vi "Dashboard Main.vi"() -> ()   [LabVIEW 2019]
uses:
  <vilib>/Utility/miscctls.llb/LVRowAndColumnTypeDef.ctl
  <vilib>/event_ctls.llb/eventvkey.ctl
  <vilib>/Rock Robotics/Network Tables/NT Read Numeric Array.vi
  <vilib>/Rock Robotics/WPI/Dashboard/WPI_DashboardLogging Global.vi
  <vilib>/Rock Robotics/Network Tables/NT Read Boolean.vi
panel:
  in  "Camera Settings Right":T1={"Frame Rate"=30, "Compression"=30, "Size"=1, "DB Camera Config"=FALSE} {"Frame Rate" scale=1.0..30.0; "Compression" scale=100.0..-1.0; "Size" items=["640x480", "320x240", "160x120"]}
  in  "Camera Name Right":string(combo)="No Camera Selection"
  out "Camera Perf":string
  in  "Camera Settings":T1={"Frame Rate"=30, "Compression"=30, "Size"=1, "DB Camera Config"=FALSE} {"Frame Rate" scale=1.0..30.0; "Compression" scale=100.0..-1.0; "Size" items=["640x480", "320x240", "160x120"]}
  in  "TCP":refnum<k5>
  in  "Rec Mode":enum32{"Stop", "Record", "Playback"}(radio)
  out "Robot IP":string
  out "Image Message":string="Timeout in Camera Communications"
  in  "Dashboard Tab":T2(tab)
  in  "Select Auto":string(combo)="Select Autonomous ..."
  out "NT Connection":bool
  out "MotorChart R":cluster{"Numeric":dbl, "Numeric":dbl}(graph)
  out "MotorChart L":cluster{"Numeric":dbl, "Numeric":dbl}(graph)
  out "MotorSliders R":cluster{"MotorSlide1":dbl, "MotorSlide2":dbl} {"MotorSlide2" scale=-1.0..1.0 scale format="%#_2e"; "MotorSlide1" scale=-1.0..1.0 scale format="%#_2e"}
  out "MotorSliders L":cluster{"MotorSlide1":dbl, "MotorSlide2":dbl} {"MotorSlide2" scale=-1.0..1.0 scale format="%#_2e"; "MotorSlide1" scale=-1.0..1.0 scale format="%#_2e"}
  out "Gyro":dbl(knob) scale=0.0..360.0
  out "JS1 Z":dbl(slide) scale=-1.0..1.0 scale format="%#_2e"
  out "JS1 Graph":cluster{"X":dbl, "Y":dbl}[](graph)
  out "JS1 Buttons":T3
  out "JS2 Z":dbl(slide) scale=-1.0..1.0 scale format="%#_2e"
  out "JS2 Graph":cluster{"X":dbl, "Y":dbl}[](graph)
  out "JS2 Buttons":T3
  out "Mode":T4(ring)=enum."Auto Disabled"
  out "Right Camera Perf":cluster{"Bandwidth (Mbps)":dbl, "FPS":dbl}
  out "Ball Intake":dbl
  out "Camera Image Right":T5(plugin-control)
  in  "DB/String 9":string
  in  "DB/String 8":string
  in  "DB/String 7":string
  in  "DB/String 6":string
  in  "DB/String 5":string
  in  "DB/String 4":string
  in  "DB/String 3":string
  in  "DB/String 2":string
  in  "DB/String 1":string
  in  "DB/String 0":string
  in  "DB/Slider 0":dbl(slide) scale=0.0..5.0
  in  "DB/Slider 1":dbl(slide) scale=0.0..5.0
  in  "DB/Slider 2":dbl(slide) scale=0.0..5.0
  in  "DB/Slider 3":dbl(slide) scale=0.0..5.0
  out "DB/LED 3":bool
  out "DB/LED 2":bool
  out "DB/LED 1":bool
  out "DB/LED 0":bool
  in  "DB/Button 3":bool
  in  "DB/Button 2":bool
  in  "DB/Button 1":bool
  in  "DB/Button 0":bool caption="New Name"
  out "Touching?":bool
  out "Color":u32(colorbox)
  out "Color Name":string
  out "Proximity":dbl
  out "Confidence":dbl
  in  "Test Slider":dbl(slide) scale=0.0..100.0 scale format="%#_3g"
  in  "On/Off":bool caption="Solenoid"
  in  "Test Name":u16(ring) items=["Select the test to run..."]
  in  "Test Tree":string(tree)
  in  "Motor":cluster{"Value":dbl, "Enable":bool} {"Value" scale=-1.0..1.0 scale format="%#_3g"}
  out "Progress":T6 {"Test Progress" scale=0.0..100.0}
  in  "Rev/Fwd":cluster{"Forward":bool, "Reverse":bool}
  in  "Test Ring":u16(ring) items=["Monochrome", "Color"]
  out "Cmd Status":string
  in  "Execute Command":bool
  in  "Command Params":string[][](table)
  in  "Command Selection":i32(listbox)
  in  "CheckList":i32(listbox)
  out "Tree":string(tree)
  out "Camera Image":T5(plugin-control)
  out "Background":bool
  in  "Camera Name":string(combo)="No Camera Selection"
  # "HW"
  # "HW"
  # "Joysticks"
  # "Drive Motors"
  # "Front"
  # "Right"
  # "Left"
  # "Back"
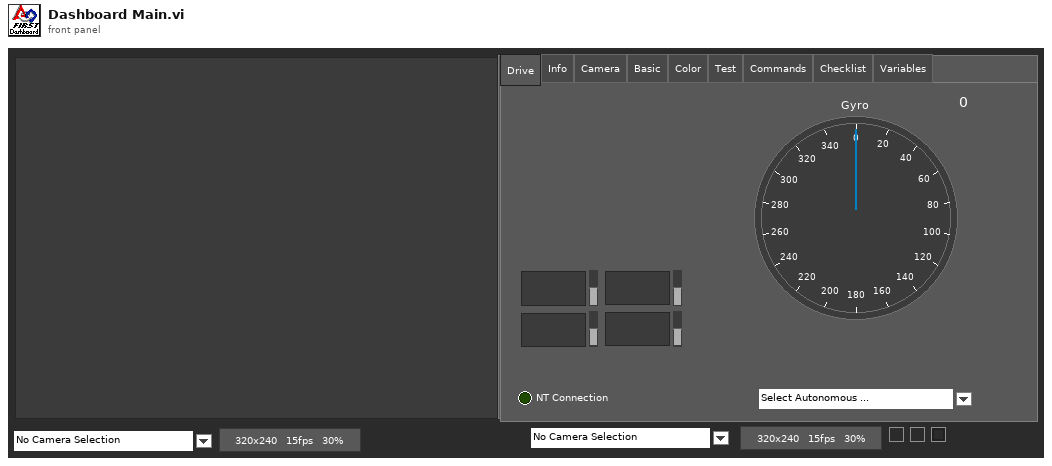
[diagram p1: front panel]
types:
  T1 = cluster{"Frame Rate":i32, "Compression":i32, "Size":u16, "DB Camera Config":bool}
  T2 = enum32{"Drive", "Info", "Camera", "Basic", "Color", "Test", "Commands", "Checklist", "Variables"}
  T3 = cluster{bool, bool, bool, bool, bool, bool, bool, bool, bool, bool, bool, bool}
  T4 = enum8{"Tele-Op Disabled", "Tele-Op Enabled", "Auto Disabled", "Auto Enabled", "Test Disabled", "Test Enabled", "Disconnected", "No Code", "E-Stop"}
  T5 = typedef "IMAQ Image.ctl" = refnum<image>
  T6 = cluster{"Test Progress":u8, "Test Progress Text":string}
  T7 = cluster{"Save Path":path, "Interval (s)":dbl, "Keep":i32}
  T8 = enum32{"Drive", "Camera", "Basic", "Custom", "Test", "Commands", "Checklist", "Variables"}
  T9 = typedef "Image Type" = u32
  T10 = cluster{"IDs":cluster{"RPC field ID":u16, "Unique ID":u16}, "String":string}
  T11 = cluster{"Error Strings":string, "Disable Counts":cluster{u16, u16}, "Rail Faults":cluster{u16, u16, u16}, "Robot IP":string, "DB Mode":u8, "Event Info":cluster{"Name":string, "Type":u8, "Number":u16, "Replay":u8}}
  T12 = cluster{"Storage":cluster{"Disk Free":u64, "RAM Block":u32, "RAM free":u32}, "CPU Utilization":cluster{"CPU % ISR":sgl, "CPU % Time Crit":sgl, "CPU % Timed Str":sgl, "CPU % High":sgl, "CPU % Above":sgl, "CPU % Normal":sgl, "CPU % Low":sgl}, "CAN":cluster{"% Bus Utilization":sgl, "Bus Off Cnt":u32, "TX_FIFO Full Cnt":u32, "Receive Error Cnt":u8, "Transmit Error Cnt":u8}, "HID":cluster{"HID Outputs":u32, "Rumble Low":u16, "Rumble High":u16}[]}
  T13 = cluster{"Status bits":cluster{"Test Mode":bool, "Autonomous":bool, "Enabled":bool, "Code Start":bool, "Brownout":bool, "Reserved 2":bool, "Reserved 3":bool, "E-Stop":bool}, "Code Trace":cluster{"Disabled":bool, "TeleOp":bool, "Auto":bool, "Test":bool}, "Controller Type":enum16{"unknown", "cRIO", "roboRio"}, "Code?":enum16{"unknown", "noCode", "code"}, "Battery V":dbl}
  T14 = cluster{"Control Bits":cluster{"TestMode":bool, "Autonomous":bool, "Enabled":bool, "FMS Present":bool, bool, bool, bool, "E-Stop":bool}, "Team Station ":u8, "Countdown":sgl, "Joystick Values":cluster{"Axes":dbl[], "Buttons":bool[], "POVs":i16[]}[]}
  T15 = cluster{"Axes":dbl[], "Buttons":bool[], "POVs":i16[]}[]
  T16 = cluster{"Axes":dbl[], "Buttons":bool[], "POVs":i16[]}
  T17 = cluster{"Buttons[0]":bool, "Buttons[1]":bool, "Buttons[2]":bool, "Buttons[3]":bool, "Buttons[4]":bool, "Buttons[5]":bool, "Buttons[6]":bool, "Buttons[7]":bool, "Buttons[8]":bool, "Buttons[9]":bool, "Buttons[10]":bool, "Buttons[11]":bool}
  T18 = cluster{"Camera Image":refnum<vi>, "Dashboard Tab":refnum<vi>, "Background":refnum<vi>, "Rec Mode":refnum<vi>, "Test Slider":refnum<vi>, "On/Off ":refnum<vi>, "Test Ring":refnum<vi>, "Rev/Fwd":refnum<vi>, "Test Name":refnum<vi>, "Motor":refnum<vi>, "Progress":refnum<vi>, "CheckList":refnum<vi>, "Tree":refnum<vi>, "Test Tree":refnum<vi>, "Command Params":refnum<vi>, "Command Selection":refnum<vi>, "Execute Command":refnum<vi>, "Cmd Status":refnum<vi>, "Camera Settings":refnum<vi>, "Camera Name":refnum<vi>, "Camera Perf":refnum<vi>, "Camera Settings Right":refnum<vi>, "Camera Name Right":refnum<vi>, "Camera Image Right":refnum<vi>}
  T19 = cluster{"Global Rectangle":i32[], "Contours":cluster{"Contour Type":u32, "ROI Type":u32, "Points":i32[]}[]}
  T20 = cluster{"Camera Name":string, string, "Saved DB Images Info":cluster{"Save Path":path, "Interval (s)":dbl, "Keep":i32}}
  T21 = cluster{"Camera Name Right":string, string, "Saved DB Images Info":cluster{"Save Path":path, "Interval (s)":dbl, "Keep":i32}}
  T22 = cluster{"Operation":enum16{"Update", "Clear"}, "Color Box":u32}[]
  T23 = typedef "eventvkey.ctl" = enum16{"ASCII", "Enter", "Return", "Shift", "Ctrl", "Alt", "Cmd", "Opt", "Caps", "NumLock", "Clear", "Break", "Up", "Down", "Left", "Right", "Insert", "Delete", "Home", "End", "PageUp", "PageDown", "Escape", "Help", "Pause", "ScrollLock", "F1", "F2", "F3", "F4", "F5", "F6", "F7", "F8", "F9", "F10", "F11", "F12", "F13", "F14", "F15", "F16", "F17", "F18", "F19", "F20", "F21", "F22", "F23", "F24", "Play", "VolumeUp", "VolumeDown", "Mute", "Two Byte Char"}
  T24 = cluster{"Image Size":bool, "Image Type":bool, "Pixel Value":bool, "ROI Information":bool, "Zoom Factor":bool}
  T25 = cluster{"Operation":enum16{"Update", "Clear"}, "Color Box":u32}
  T26 = typedef "LVRowAndColumnTypeDef.ctl" = cluster{"Row":i32, "Column":i32}
  T27 = cluster{"Shift":bool, "Ctrl":bool, "Alt":bool, "Cmd":bool, "Opt":bool}
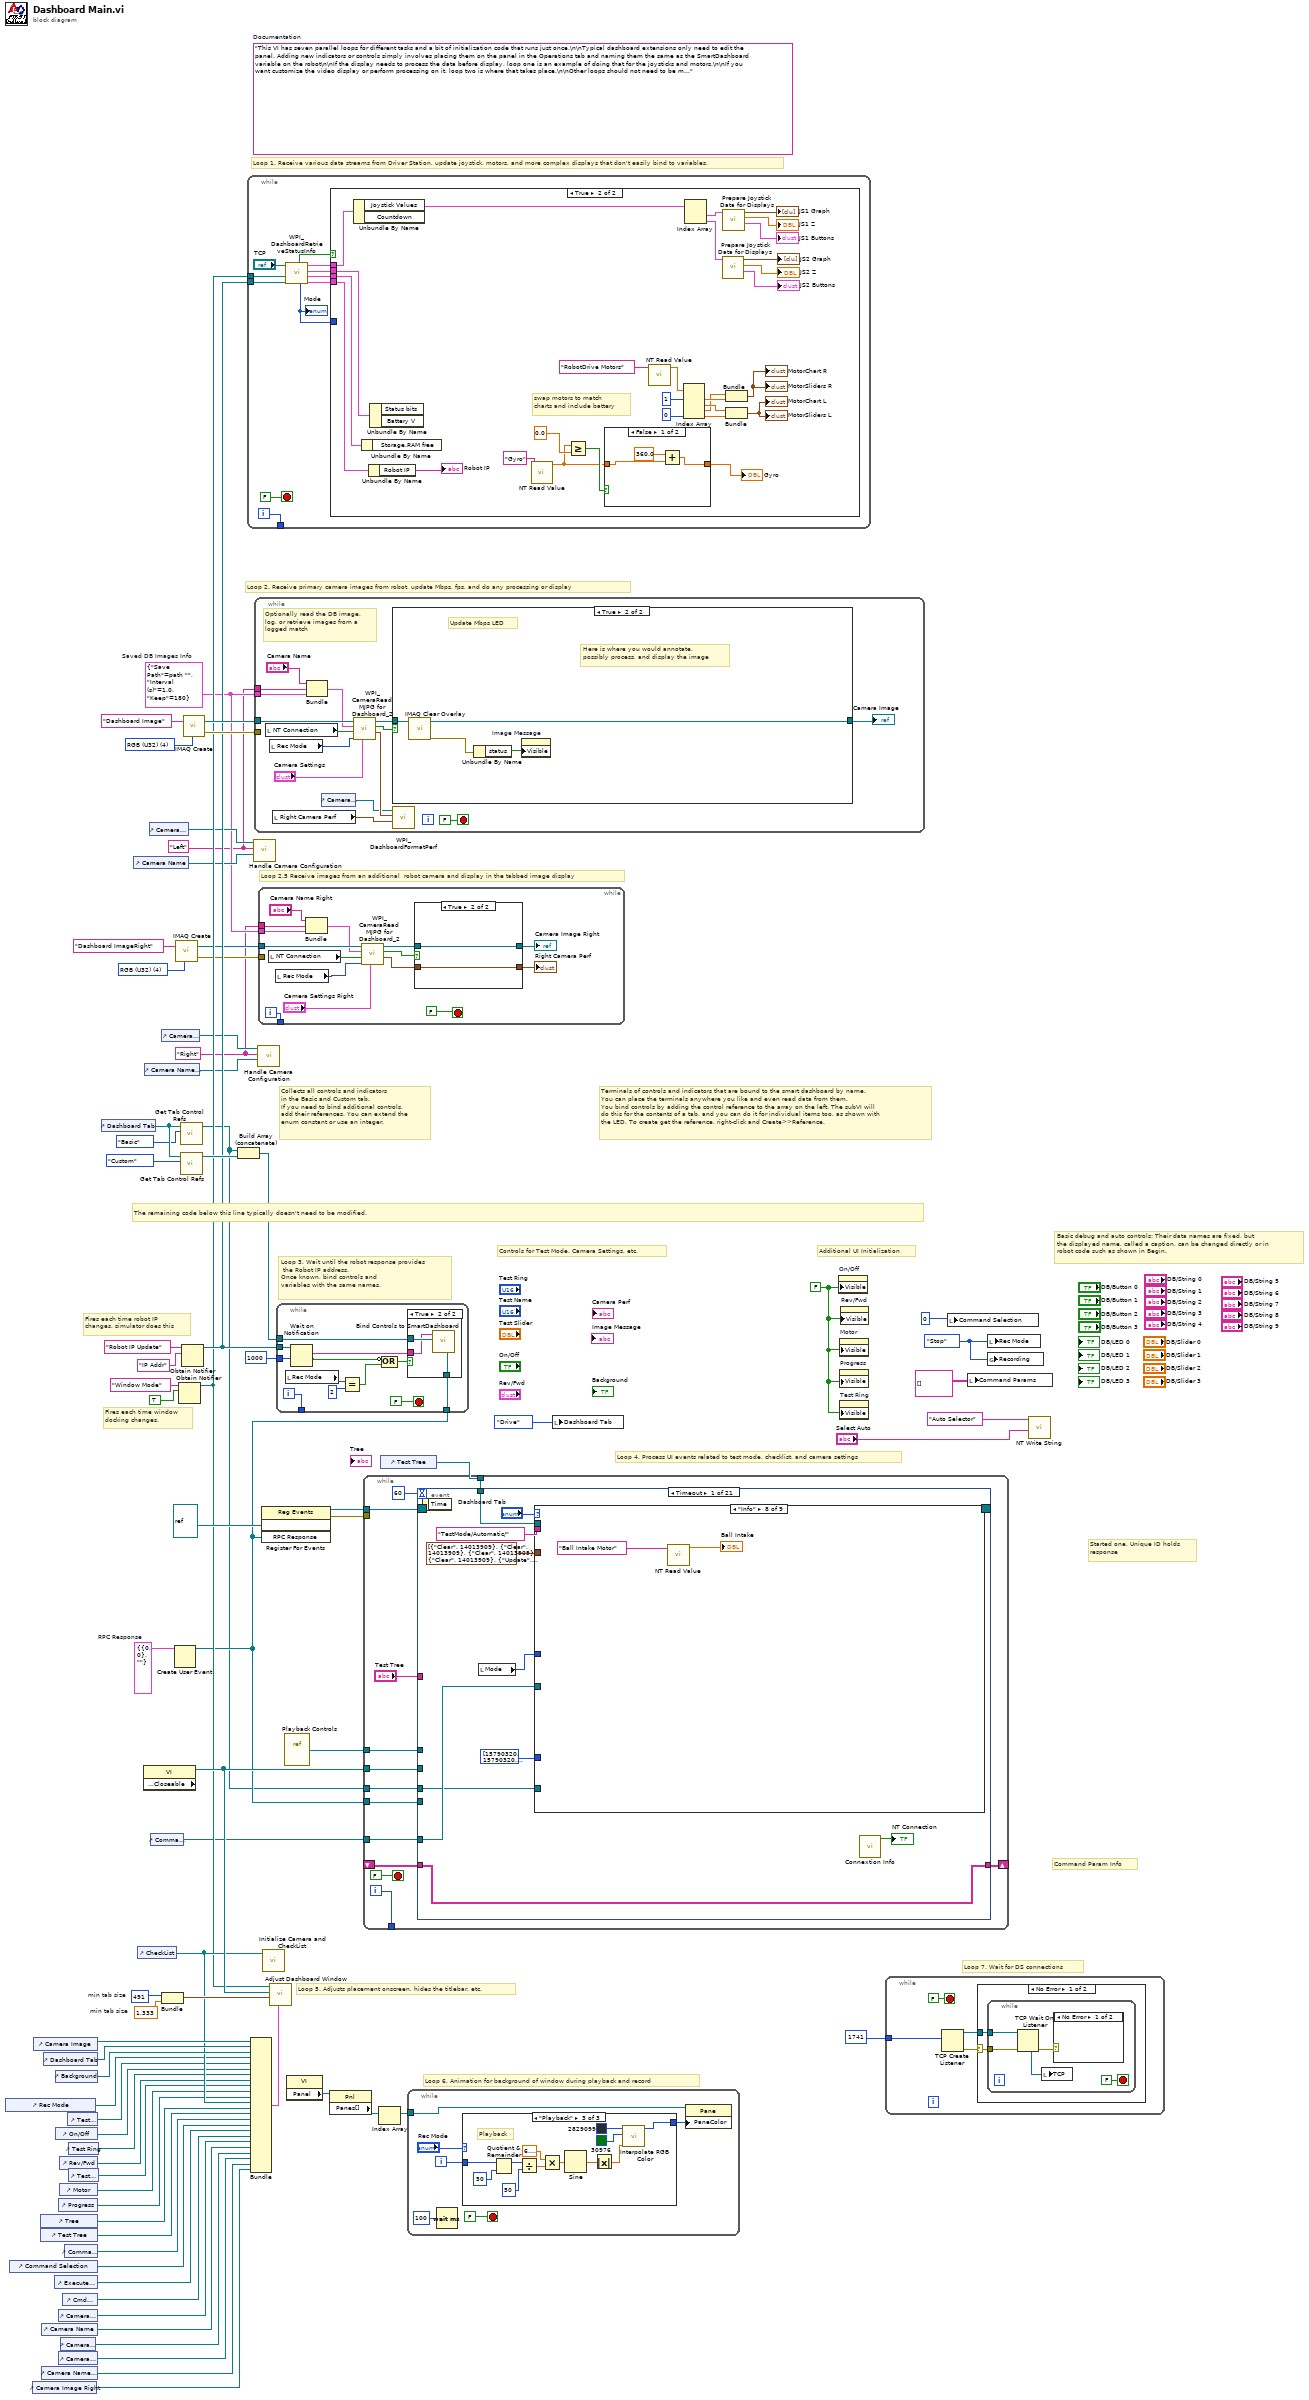
[diagram p0: block diagram]
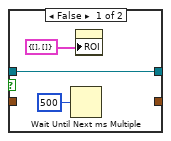
[diagram p2: hidden frame]
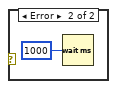
[diagram p3: hidden frame]
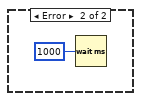
[diagram p4: hidden frame]
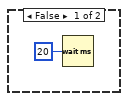
[diagram p5: hidden frame]
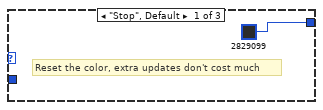
[diagram p7: hidden frame]
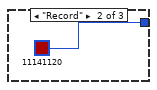
[diagram p8: hidden frame]
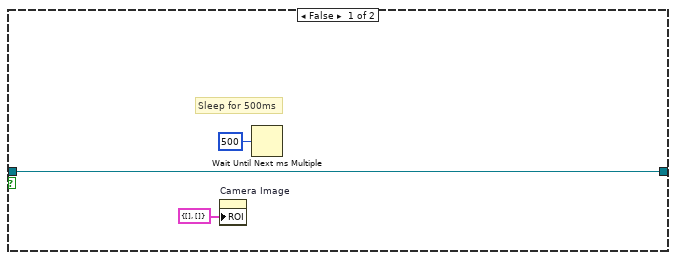
[diagram p10: hidden frame]
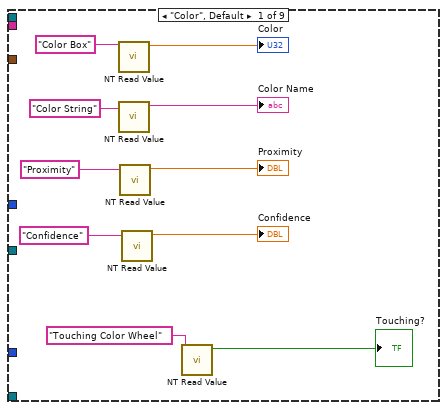
[diagram p11: hidden frame]
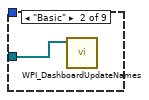
[diagram p12: hidden frame]
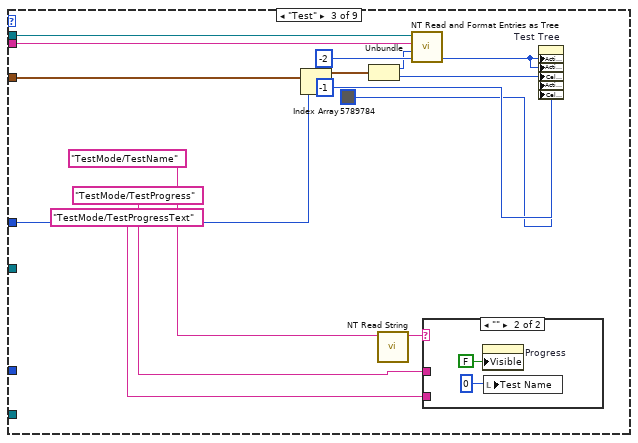
[diagram p13: hidden frame]
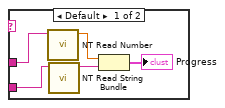
[diagram p14: hidden frame]
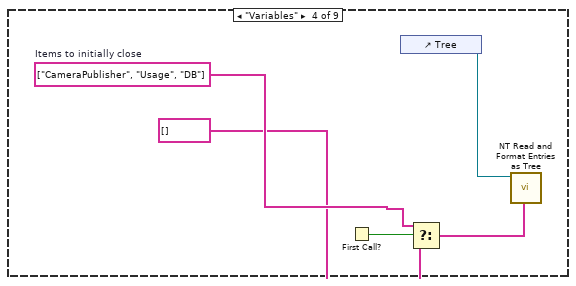
[diagram p15: hidden frame]
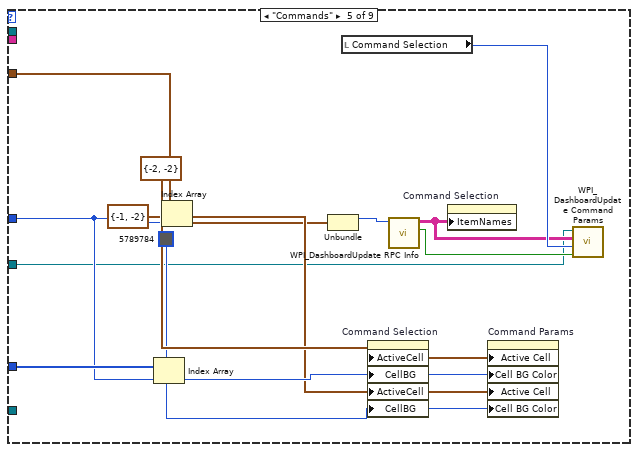
[diagram p16: hidden frame]
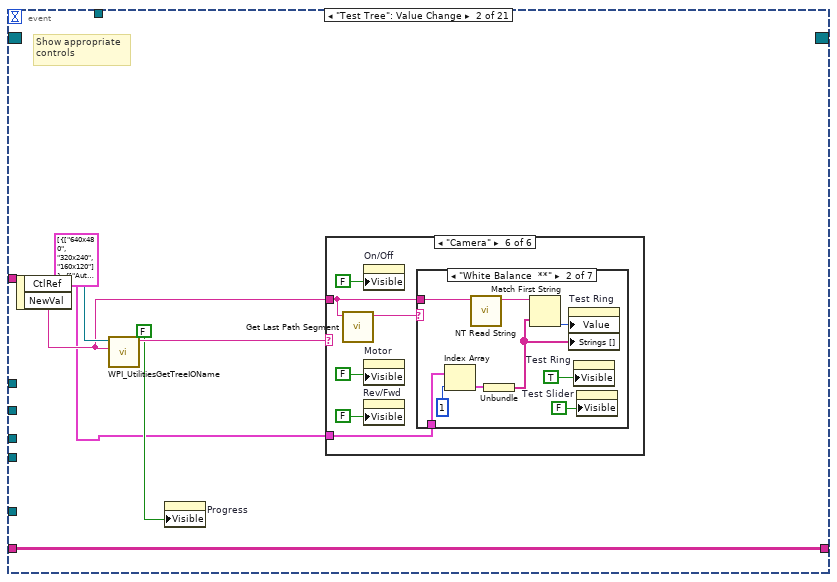
[diagram p20: hidden frame]
diagram:
  w3 = T7 {"Save Path"=path "", "Interval (s)"=1.0, "Keep"=180}  # Saved DB Images Info
  w2 = "Right"
  w1 = "Left"
  w13 = T9 4 items=["Grayscale (U8)", "Grayscale (I16)", "Grayscale (SGL)", "Complex (CSG)", "RGB (U32)", "HSL (U32)", "RGB (U64)"] ("Image Type")
  w29 = T10 {"IDs"={"RPC field ID"=0, "Unique ID"=0}, "String"=""}  # RPC Response
  w52 = 491  # min tab size
  w51 = 1.333  # min tab size
  w59 = enum32{"Stop", "Record", "Playback"}."Stop" ("Rec Mode")
  w36 = FALSE ("Visible")
  (unwired) "This VI has seven parallel loops for different tasks and a bit of initialization code that runs just once.\n\nTypical dashboard extensions only need to edit the panel. Adding new indicators or controls simply involves placing them on the panel in the Operations tab and naming them the same as the SmartDashboard variable on the robot\n\nIf the display needs to process the data before display, loop one is an example of doing that for the joysticks and motors.\n\nIf you want customize the video display or perform processing on it, loop two is where that takes place.\n\nOther loops should not need to be modified. They are pretty standard, and document the task they perform."  # Documentation
  w76 = T9 4 items=["Grayscale (U8)", "Grayscale (I16)", "Grayscale (SGL)", "Complex (CSG)", "RGB (U32)", "HSL (U32)", "RGB (U64)"] ("Image Type")
  # "Loop 2.5 Receive images from an additional  robot camera and display in the tabbed image display"
  # "Command Param Info"
  # "Started one, Unique ID holds\nresponse"
  # "Loop 7. Wait for DS connections"
  # "Basic debug and auto controls: Their data names are fixed, but\nthe displayed name, called a caption, can be changed directly or in\nrobot code such as shown in Begin."
  # "Controls for Test Mode, Camera Settings, etc."
  # "Additional UI Initialization"
  # "Loop 6. Animation for background of window during playback and record"
  # "Fires each time robot IP\nchanges, simulator does this"
  # "Fires each time window\ndocking changes."
  # "Collects all controls and indicators\nin the Basic and Custom tab.\nIf you need to bind additional controls,\nadd their references. You can extend the\nenum constant or use an integer."
  # "The remaining code below this line typically doesn't need to be modified."
  # "Loop 4. Process UI events related to test mode, checklist, and camera settings"
  # "Terminals of controls and indicators that are bound to the smart dashboard by name.\nYou can place the terminals anywhere you like and even read data from them.\nYou bind controls by adding the control reference to the array on the left. The subVI will\ndo this for the contents of a tab, and you can do it for individual items too, as shown with\nthe LED. To create get the reference, right-click and Create>>Reference."
  # "Loop 3. Wait until the robot response provides\n the Robot IP address.\nOnce known, bind controls and\nvariables with the same names."
  # "Loop 5. Adjusts placement onscreen, hides the titlebar, etc."
  # "Loop 1. Receive various data streams from Driver Station, update joystick, motors, and more complex displays that don't easily bind to variables."
  # "Loop 2. Receive primary camera images from robot, update Mbps, fps, and do any processing or display"
  n1 = control-ref of="Rec Mode"() -> (w42:refnum<vi>)
  n2 = control-ref of="Command Selection"() -> (w28:refnum<vi>)
  n3 = control-ref of="Camera Image Right"() -> (w6:refnum<vi>)
  n4 = control-ref of="Camera Image"() -> (w54:refnum<vi>)
  n5 = control-ref of="Tree"() -> (w46:refnum<vi>)
  n6 = control-ref of="Test Tree"() -> (w45:refnum<vi>)
  n7 = control-ref of="Camera Name"() -> (w19:refnum<vi>)
  n8 = control-ref of="Camera Name Right"() -> (w7:refnum<vi>)
  n9 = control-ref of="Dashboard Tab"() -> (w53:refnum<vi>)
  n10 = control-ref of="Execute Command"() -> (w30:refnum<vi>)
  n11 = control-ref of="Background"() -> (w49:refnum<vi>)
  n12 = control-ref of="On/Off"() -> (w40:refnum<vi>)
  n13 = control-ref of="Progress"() -> (w37:refnum<vi>)
  n14 = control-ref of="Camera Settings"() -> (w20:refnum<vi>)
  n15 = control-ref of="Camera Settings Right"() -> (w8:refnum<vi>)
  n16 = control-ref of="Rev/Fwd"() -> (w38:refnum<vi>)
  n17 = control-ref of="Motor"() -> (w43:refnum<vi>)
  n18 = control-ref of="Camera Perf"() -> (w18:refnum<vi>)
  n19 = control-ref of="Cmd Status"() -> (w24:refnum<vi>)
  n20 = control-ref of="Command Params"() -> (w31:refnum<vi>)
  n21 = control-ref of="Test Slider"() -> (w41:refnum<vi>)
  n22 = control-ref of="Test Ring"() -> (w39:refnum<vi>)
  n23 = control-ref of="Test Name"() -> (w44:refnum<vi>)
  n24 = control-ref of="Dashboard Tab"() -> (w57:refnum<vi>)
  n25 = control-ref of="Camera Name"() -> (w21:refnum<vi>)
  n26 = control-ref of="CheckList"() -> (w47:refnum<vi>)
  n27 = property class="VI" props=["Front Panel.Closeable"]() -> (reference out=w58:refnum<vi>)  [unwired: 2 in, 2 out]
  n28 = control-ref of="Camera Name Right"() -> (w9:refnum<vi>)
  n29 = control-ref of="Camera Settings"() -> (w22:refnum<vi>)
  n30 = control-ref of="Command Params"() -> (w23:refnum<vi>)
  n31 = control-ref of="Camera Settings Right"() -> (w10:refnum<vi>)
  n32 = Bundle("min tab size"=w52, "min tab size"=w51) -> (w50:cluster{"min tab size":i32, "min tab size":dbl})  [unwired: 1 in]
  n33 = Create User Event(user event datatype=w29) -> (user event=w25:refnum<user-event>)  [unwired: 1 in, 1 out]
  n34 = call "IMAQ Create"("Image Name"="Dashboard ImageRight", "Image Type"=w13) -> ("New Image"=w12:T5, "error out"=w11:errorcluster)  [unwired: 2 in, 1 out]
  n35 = Obtain Notifier(name (unnamed)="Window Mode", notification data type=TRUE) -> (notifier out=w34:refnum<notifier>)  [unwired: 2 in, 2 out]
  n36 = call <vilib>:"Get Tab Control Refs.vi"("Page Index"=T8."Basic" ("Dashboard Tab"), "TabControl in"=w57) -> ("ControlsOnPage"=w17:refnum<vi>[])  [unwired: 9 in]
  n37 = call <vilib>:"Get Tab Control Refs.vi"("Page Index"=T8."Custom" ("Dashboard Tab"), "TabControl in"=w57) -> ("ControlsOnPage"=w56:refnum<vi>[])  [unwired: 9 in]
  n38 = Obtain Notifier(name (unnamed)="Robot IP Update", notification data type="IP Addr" ("name (unnamed)")) -> (notifier out=w35:refnum<notifier>)  [unwired: 2 in, 2 out]
  n39 = call "IMAQ Create"("Image Name"="Dashboard Image", "Image Type"=w76) -> ("New Image"=w74:T5, "error out"=w73:errorcluster)  [unwired: 2 in, 1 out]
  n40 = Build Array (concatenate)(w17, w56) -> (w55:refnum<vi>[])
  n41 = while {
    tunnel: [w86] -> _
    tunnel: w35 -> [w80]
    tunnel: w34 -> [w77]
    i -> [w86]
    stop <- FALSE stop-if-true
    n42 = call <vilib>:"WPI_DashboardRetrieveStatusInfo.vi"("Binding Refnum"=w80, "Window Mode Notifier"=w77, "TCP Cnx"="TCP") -> ("Power and Errors"=w81:T11, "Robot Metrics"=w84:T12, "Status Info"=w85:T13, "Control Info"=w82:T14, "Robot Mode"=w79:T4, "Process?"=w83:bool)  [unwired: 3 in]
    "Mode" <- w79
    n43 = case shown="True" w83 {
      tunnel: w85 -> [_ w117]
      tunnel: w84 -> [_ w116]
      tunnel: w82 -> [_ w115]
      tunnel: w81 -> [_ w114]
      tunnel: w79 -> [_ _]
      frame False {
        n44 = Wait (ms)(milliseconds to wait=u32 20) -> ()  [unwired: 1 out]
      }
      frame True {
        # "swap motors to match\ncharts and include battery"
        n45 = Unbundle By Name(w115) -> ("Joystick Values"=w105:T15)  [unwired: 1 out]
        n46 = Unbundle By Name(w116) -> ()  [unwired: 1 out]
        n47 = Unbundle By Name(w114) -> ("Robot IP"=→"Robot IP":string)
        n48 = Unbundle By Name(w117) -> ()  [unwired: 2 out]
        n49 = call-poly <vilib>:"NT Read Value.vi"("Name"="Gyro") -> ("Numeric"=w90:dbl)  [unwired: 9 in, 1 out]
        n50 = Greater Or Equal?(x=w90, y=0.0) -> (x >= y?=w91:bool)
        n51 = case shown="False" w91 {
          tunnel: w90 -> [w120 w121]
          tunnel: [w118 w121] -> w89
          frame False {
            n52 = Add(x=360.0, y=w120) -> (x+y=w118:dbl)
          }
          frame True {
          }
        }
        "Gyro" <- w89
        n53 = call-poly <vilib>:"NT Read Value.vi"("Name"="RobotDrive Motors") -> ("Numeric Array"=w95:dbl[])  [unwired: 9 in, 1 out]
        n54 = Index Array(array=w95, index #1=1, index #4=0) -> (element #1=w109:dbl, element #2=w110:dbl, element #3=w108:dbl, element #4=w113:dbl)  [unwired: 2 in]
        n55 = Index Array(array=w105) -> (element #1=w104:T16, element #2=w100:T16)  [unwired: 2 in]
        n56 = call "Prepare Joystick Data for Displays.vi"("Joystick Values"=w100) -> ("Buttons"=→"JS2 Buttons":T17, "Z Axis"=→"JS2 Z":dbl, "Cartesian Data"=→"JS2 Graph":cluster{"X axis":dbl, "X axis":dbl}[])  [unwired: 8 in]
        n57 = call "Prepare Joystick Data for Displays.vi"("Joystick Values"=w104) -> ("Buttons"=→"JS1 Buttons":T17, "Z Axis"=→"JS1 Z":dbl, "Cartesian Data"=→"JS1 Graph":cluster{"X axis":dbl, "X axis":dbl}[])  [unwired: 8 in]
        n58 = Bundle("Numeric"=w108, "Numeric"=w109) -> (→"MotorChart R" →"MotorSliders R":cluster{"Numeric":dbl, "Numeric":dbl})  [unwired: 1 in]
        n59 = Bundle("Numeric"=w110, "Numeric"=w113) -> (→"MotorChart L" →"MotorSliders L":cluster{"Numeric":dbl, "Numeric":dbl})  [unwired: 1 in]
      }
    }
  }
  n60 = Bundle("Camera Image"=w54, "Dashboard Tab"=w53, "Background"=w49, "Rec Mode"=w42, "Test Slider"=w41, "On/Off"=w40, "Test Ring"=w39, "Rev/Fwd"=w38, "Test Name"=w44, "Motor"=w43, "Progress"=w37, "CheckList"=w47, "Tree"=w46, "Test Tree"=w45, "Command Params"=w31, "Command Selection"=w28, "Execute Command"=w30, "Cmd Status"=w24, "Camera Settings"=w20, "Camera Name"=w19, "Camera Perf"=w18, "Camera Settings Right"=w8, "Camera Name Right"=w7, "Camera Image Right"=w6) -> (w48:T18)  [unwired: 1 in]
  n61 = call "Handle Camera Configuration.vi"("CameraNameRef"=w21, "Display Name"=w1, "ClusterRef"=w22) -> ()  [unwired: 9 in]
  n62 = while {
    tunnel: w74 -> [w135]
    tunnel: w73 -> [_]
    tunnel: w3 -> [w128]
    tunnel: w1 -> [w125]
    stop <- FALSE stop-if-true
    # "Optionally read the DB image,\nlog, or retrieve images from a\nlogged match"
    n63 = local read "NT Connection"() -> (w129:bool)
    n64 = local read "Rec Mode"() -> (w132:enum32{"Stop", "Record", "Playback"})
    n65 = local read "Right Camera Perf"() -> (w123:cluster{"Bandwidth (Mbps)":dbl, "FPS":dbl})
    n66 = Bundle("Camera Name"="Camera Name", w125, "Saved DB Images Info"=w128) -> (w127:T20)  [unwired: 1 in]
    n67 = control-ref of="Camera Perf"() -> (w122:refnum<vi>)
    n68 = call <vilib>:"WPI_CameraRead MJPG for Dashboard_2.vi"("Camera Settings"="Camera Settings", "Rec Mode"=w132, "NT Connection"=w129, "Capture Info"=w127, "Image in"=w135) -> ("perf info"=w124:cluster{"Bandwidth (Mbps)":dbl, "fps":dbl}, "Active"=w133:bool, "Image\\ out"=w134:T5)  [unwired: 4 in]
    n69 = case shown="True" w133 {
      tunnel: w134 -> [w138 w141]
      tunnel: [w138 w140] -> w130
      frame False {
        # "Sleep for 500ms"
        n70 = property on="Camera Image" class="ImageControl"("ROI"=T19 {"Global Rectangle"=[], "Contours"=[]}) -> ()  [unwired: 2 in, 2 out]
        n71 = Wait Until Next ms Multiple(millisecond multiple=u32 500) -> ()  [unwired: 1 out]
      }
      frame True {
        # "Here is where you would annotate,\npossibly process, and display the image"
        # "Update Mbps LED"
        n72 = call "IMAQ Clear Overlay"("Image"=w141) -> ("error out"=w142:errorcluster, "Image Out"=w140:T5)  [unwired: 2 in, 7 out]
        n73 = Unbundle By Name(w142) -> ("status"=w143:bool)
        n74 = property on="Image Message" class="Str"("Visible"=w143) -> ()  [unwired: 2 in, 2 out]
      }
    }
    "Camera Image" <- w130
    n75 = call <vilib>:"WPI_DashboardFormatPerf.vi"("Right Camera Perf"=w123, "Performance"=w124, "String in"=w122) -> ()  [unwired: 9 in]
  }
  n76 = call "Handle Camera Configuration.vi"("CameraNameRef"=w9, "Display Name"=w2, "ClusterRef"=w10) -> ()  [unwired: 9 in]
  n77 = while {
    tunnel: w12 -> [w158]
    tunnel: w11 -> [_]
    tunnel: [w153] -> _
    tunnel: w3 -> [w149]
    tunnel: w2 -> [w146]
    i -> [w153]
    stop <- FALSE stop-if-true
    n78 = local read "NT Connection"() -> (w150:bool)
    n79 = local read "Rec Mode"() -> (w157:enum32{"Stop", "Record", "Playback"})
    n80 = Bundle("Camera Name Right"="Camera Name Right", w146, "Saved DB Images Info"=w149) -> (w148:T21)  [unwired: 1 in]
    n81 = call <vilib>:"WPI_CameraRead MJPG for Dashboard_2.vi"("Camera Settings"="Camera Settings Right", "Rec Mode"=w157, "NT Connection"=w150, "Capture Info"=w148, "Image in"=w158) -> ("perf info"=w144:cluster{"Bandwidth (Mbps)":dbl, "fps":dbl}, "Active"=w152:bool, "Image\\ out"=w155:T5)  [unwired: 4 in]
    n82 = case shown="True" w152 {
      tunnel: w155 -> [w160 w163]
      tunnel: [w160 w163] -> w151
      tunnel: [_ w162] -> w145
      tunnel: w144 -> [_ w162]
      frame False {
        n83 = Wait Until Next ms Multiple(millisecond multiple=u32 500) -> ()  [unwired: 1 out]
        n84 = property on="Camera Image Right" class="ImageControl"("ROI"=T19 {"Global Rectangle"=[], "Contours"=[]}) -> ()  [unwired: 2 in, 2 out]
      }
      frame True {
      }
    }
    "Camera Image Right" <- w151
    "Right Camera Perf" <- w145
  }
  n85 = register-events(refnum<vi> refnum, w25) -> (reference out=w63:refnum<event-registration>, error out=w62:errorcluster)  [unwired: 2 in]
  n86 = call "Initialize Camera and CheckList.vi"("ListBox in"=w47) -> ()  [unwired: 11 in]
  n87 = call "Adjust Dashboard Window.vi"("Sizing Refnums"=w48, "Size Constraints"=w50, "VI"=w58, "WIn Mode"=w34) -> ()  [unwired: 8 in]
  n88 = while {
    tunnel: w55 -> [w175]
    tunnel: w35 -> [w173]
    tunnel: [w171] -> _
    tunnel: u32 1000 ("milliseconds to wait") -> [w170]
    tunnel: w25 -> [w164]
    i -> [w171]
    stop <- FALSE stop-if-true
    n89 = local read "Rec Mode"() -> (w166:enum32{"Stop", "Record", "Playback"})
    n90 = Wait on Notification(notifier=w173, timeout in ms (-1)=w170) -> (notification=w172:string, timed out?=w168:bool)  [unwired: 2 in, 2 out]
    n91 = Equal?(x=w166, y=u16 2 ("Rec Mode")) -> (x = y?=w167:bool)
    n92 = Compound Arithmetic op=OR(invert w168, w167) -> (w169:bool)
    n93 = case shown="True" w169 {
      tunnel: w175 -> [_ w178]
      tunnel: w172 -> [_ w177]
      tunnel: w164 -> [_ w176]
      frame False {
      }
      frame True {
        n94 = call <vilib>:"Bind Controls to SmartDashboard.vi"("RPC ref"=w176, "Bound Control Refs"=w178, "Server IP Address"=w177) -> ()  [unwired: 9 in]
      }
    }
  }
  n95 = vi-ref "Playback Controls.vi"() -> (w64:refnum<vi>)
  n96 = property class="VI"() -> ("Panel"=w66:refnum<vi>)  [unwired: 2 in, 2 out]
  n97 = property class="Pnl"(reference=w66) -> ("Panes[]"=w67:refnum<vi>[])  [unwired: 1 in, 2 out]
  n98 = Index Array(array=w67) -> (element=w65:refnum<vi>)  [unwired: 1 in]
  n99 = control-ref of="Test Tree"() -> (w68:refnum<vi>)
  n100 = while {
    tunnel: [w188] -> _
    tunnel: w68 -> [w187]
    tunnel: w64 -> [w186]
    tunnel: w63 -> [w185]
    tunnel: w62 -> [_]
    tunnel: w58 -> [w184]
    tunnel: w25 -> [w183]
    tunnel: w23 -> [w182]
    shift-right: [w181] -> _
    shift-left: _ -> [w180]
    tunnel: w17 -> [w179]
    i -> [w188]
    stop <- FALSE stop-if-true
    n101 = event shown="[0] Timeout" {
      selector: w185 -> [_ _ _ _ _ _ _ _ _ _ _ _ _ _ _ _ _ _ _ _ _]
      dyn-events: [_ _ _ _ _ _ _ _ _ _ _ _ _ _ _ _ w460 _ _ _ _] -> _
      timeout: u32 60 ("milliseconds to wait") -> [_ _ _ _ _ _ _ _ _ _ _ _ _ _ _ _ _ _ _ _ _]
      tunnel: w187 -> [w200 _ _ _ _ _ _ _ _ _ _ _ _ _ _ _ _ _ _ _ _]
      tunnel: "Test Tree" -> [_ _ _ _ _ _ _ _ _ _ _ w427 w435 w437 w441 w449 _ _ _ _ _]
      tunnel: w186 -> [_ _ _ _ _ _ _ _ _ _ _ _ _ _ _ _ w462 _ w480 _ _]
      tunnel: w184 -> [_ _ _ _ _ _ _ _ _ _ _ _ _ _ _ _ w458 _ _ _ _]
      tunnel: w183 -> [_ _ _ _ _ _ _ _ _ _ _ _ _ _ _ _ w456 _ _ _ _]
      tunnel: w182 -> [w195 _ _ _ _ _ w378 _ _ _ _ _ _ _ _ _ _ _ _ _ _]
      tunnel: [w194 w255 w357 w362 w371 w375 w376 w385 w395 w402 w414 w426 w433 w436 w440 w448 w455 w475 w477 w481 w494] -> w181
      tunnel: w180 -> [w194 w255 w357 w362 w371 w375 w376 _ _ w402 w414 w426 w433 w436 w440 w448 w455 w475 w477 w481 w494]
      tunnel: w179 -> [w192 _ _ _ _ _ _ _ _ _ _ _ _ _ _ _ _ _ _ _ _]
      event Timeout {
        n102 = event-data() -> ()  [unwired: 1 in, 1 out]
        n103 = local read "Mode"() -> (w197:T4)
        n104 = case shown="\"Info\"" "Dashboard Tab" {
          tunnel: w200 -> [_ _ w226 _ _ _ _ _ _]
          tunnel: "TestMode/Automatic/" ("Name Pattern") -> [_ _ w225 _ _ _ _ _ _]
          tunnel: T22 [{"Operation"=enum."Clear", "Color Box"=14013909}, {"Operation"=enum."Clear", "Color Box"=14013909}, {"Operation"=enum."Clear", "Color Box"=14013909}, {"Operation"=enum."Clear", "Color Box"=14013909}, {"Operation"=enum."Update", "Color Box"=14013909}, {"Operation"=enum."Update", "Color Box"=16777215}, {"Operation"=enum."Clear", "Color Box"=14013909}, {"Operation"=enum."Clear", "Color Box"=14013909}, {"Operation"=enum."Clear", "Color Box"=14013909}] -> [_ _ w218 _ w246 _ _ _ _]
          tunnel: w197 -> [_ _ w217 _ w245 _ _ _ _]
          tunnel: u32[] [15790320, 15790320, 15790320, 15790320, 16777215, 16777215, 15790320, 15790320, 15790320] -> [_ _ _ _ w251 _ _ _ _]
          tunnel: w195 -> [_ _ _ _ w239 _ _ _ _]
          tunnel: w192 -> [_ w212 _ _ _ _ _ _ _]
          frame "Color", Default {
            n105 = call-poly <vilib>:"NT Read Value.vi"("Name"="Color Box") -> ("Numeric"=→"Color":dbl)  [unwired: 9 in, 1 out]
            n106 = call-poly <vilib>:"NT Read Value.vi"("Name"="Color String") -> ("String"=→"Color Name":string)  [unwired: 9 in, 1 out]
            n107 = call-poly <vilib>:"NT Read Value.vi"("Name"="Proximity") -> ("Numeric"=→"Proximity":dbl)  [unwired: 9 in, 1 out]
            n108 = call-poly <vilib>:"NT Read Value.vi"("Name"="Confidence") -> ("Numeric"=→"Confidence":dbl)  [unwired: 9 in, 1 out]
            n109 = call-poly <vilib>:"NT Read Value.vi"("Name"="Touching Color Wheel") -> ("Boolean"=→"Touching?":bool)  [unwired: 9 in, 1 out]
          }
          frame "Basic" {
            n110 = call <vilib>:"WPI_DashboardUpdateNames.vi"("Controls on Tab"=w212) -> ()  [unwired: 11 in]
          }
          frame "Test" {
            w224 = -2 ("Active Item:Row Number")
            n111 = Index Array(array=w218, index=w217) -> (element=w219:T25)
            n112 = Unbundle(w219) -> ("Operation"=w220:enum16{"Update", "Clear"}, "Color Box"=w221:u32)
            n113 = call <vilib>:"NT Read String.vi"("Name"="TestMode/TestName") -> ("String"=w215:string)  [unwired: 9 in, 1 out]
            n114 = call <vilib>:"NT Read and Format Entries as Tree.vi"("Operation"=w220, "Name Pattern"=w225, "Tree Refnum"=w226) -> ()  [unwired: 7 in, 2 out]
            n115 = case shown="\"\"" w215 {
              tunnel: "TestMode/TestProgress" ("Name") -> [w228 _]
              tunnel: "TestMode/TestProgressText" ("Name") -> [w227 _]
              frame Default {
                n116 = call <vilib>:"NT Read Number.vi"("Name"=w228) -> ("Numeric"=w229:dbl)  [unwired: 9 in, 1 out]
                n117 = call <vilib>:"NT Read String.vi"("Name"=w227) -> ("String"=w230:string)  [unwired: 9 in, 1 out]
                n118 = Bundle("Numeric"=w229, "String"=w230) -> (→"Progress":cluster{"Numeric":dbl, "String":string})  [unwired: 1 in]
              }
              frame "" {
                n119 = property on="Progress" class="Clust (strict)"("Visible"=FALSE) -> ()  [unwired: 2 in, 2 out]
                n120 = local write "Test Name"(u16 0) -> ()
              }
            }
            n121 = property on="Test Tree" class="Tree (strict)"("Active Item Row Number"=w224, "ActiveColNum"=w224, "CellBG"=w221, "Active Item Row Number"=-1 ("Active Item:Row Number"), "CellBG"=u32 5789784 ("Color Box")) -> ()  [unwired: 2 in, 2 out]
          }
          frame "Variables" {
            w236 = string[] ["CameraPublisher", "Usage", "DB"]  # Items to initially close
            n122 = First Call?() -> (First Call?: T/F=w237:bool)
            n123 = control-ref of="Tree"() -> (w238:refnum<vi>)
            n124 = Select(t=w236, s=w237, f=string[] []) -> (s? t:f=w234:string[])
            n125 = call <vilib>:"NT Read and Format Entries as Tree.vi"("Tags to  Close"=w234, "Tree Refnum"=w238) -> ()  [unwired: 8 in, 2 out]
          }
          frame "Commands" {
            w247 = u32 5789784 ("Color Box")
            w248 = T26 {"Row"=-1, "Column"=-2} ("Active Cell:Active Cell")
            w250 = T26 {"Row"=-2, "Column"=-2} ("Active Cell:Active Cell")
            n126 = Index Array(array=w251, index=w245) -> (element=w249:u32)
            n127 = Index Array(array=w246, index=w245) -> (element=w244:T25)
            n128 = Unbundle(w244) -> ("Operation"=w243:enum16{"Update", "Clear"})  [unwired: 1 out]
            n129 = local read "Command Selection"() -> (w242:i32)
            n130 = property on="Command Selection" class="MCListbox (strict)"("ActiveCell"=w250, "CellBG"=w249, "ActiveCell"=w248, "CellBG"=w247) -> ()  [unwired: 2 in, 2 out]
            n131 = call <vilib>:"WPI_DashboardUpdate RPC Info.vi"("Operation"=w243) -> ("update"=w241:bool, "commands"=w240:string[][])  [unwired: 9 in]
            n132 = property on="Command Selection" class="MCListbox (strict)"("ItemNames"=w240) -> ()  [unwired: 2 in, 2 out]
            n133 = property on="Command Params" class="Tbl (strict)"("Active Cell"=w250, "Cell BG Color"=w249, "Active Cell"=w248, "Cell BG Color"=w247) -> ()  [unwired: 2 in, 2 out]
            n134 = call <vilib>:"WPI_DashboardUpdate Command Params.vi"("Update"=w241, "NewVal"=w242, "Commands"=w240, "Param Tbl"=w239) -> ()  [unwired: 7 in, 1 out]
          }
          frame "Checklist" {
          }
          frame "Camera" {
          }
          frame "Info" {
            n135 = call-poly <vilib>:"NT Read Value.vi"("Name"="Ball Intake Motor") -> ("Numeric"=→"Ball Intake":dbl)  [unwired: 9 in, 1 out]
          }
          frame "Drive" {
          }
        }
        n136 = call <vilib>:"Connextion Info.vi"() -> ("Connected"=→"NT Connection":bool)  [unwired: 10 in, 1 out]
      }
      event "Test Tree": Value Change {
        # "Show appropriate\ncontrols"
        n137 = event-data() -> ("CtlRef"=w258:refnum<vi>, "NewVal"=w256:string)  [unwired: 1 in]
        n138 = call <vilib>:"WPI_UtilitiesGetTreeIOName.vi"("NewVal"=w256, "TreeControl in"=w258) -> ("I/O Name"=w259:string)  [unwired: 9 in]
        n139 = property on="Progress" class="Clust (strict)"("Visible"=FALSE) -> ()  [unwired: 2 in, 2 out]
        n140 = case shown="\"Camera\"" w259 {
          selector: w259 -> [_ w266 _ w288 w297 _]
          tunnel: w256 -> [_ _ w285 w287 _ w304]
          tunnel: cluster{string[]}[] [{["640x480", "320x240", "160x120"]}, {["Auto", "Fixed indoor", "Fixed outdoor 1", "Fixed outdoor 2", "Fixed fluorescent 1", "Fixed fluorescent 2", "Hold current"]}, {["Auto", "Flicker-free 50 Hz", "Flicker-free 60 Hz", "Hold current"]}, {["None", "Prioritize frame rate", "Prioritize image quality"]}, {["Monochrome", "Color"]}] -> [_ _ _ _ _ w303]
          frame Default {
            w261 = FALSE ("Visible")
            w260 = FALSE ("Visible")
            n141 = property on="Motor" class="Clust (strict)"("Visible"=w260) -> ()  [unwired: 2 in, 2 out]
            n142 = property on="Test Ring" class="Ring (strict)"("Visible"=w260) -> ()  [unwired: 2 in, 2 out]
            n143 = property on="Rev/Fwd" class="Clust (strict)"("Visible"=w261) -> ()  [unwired: 2 in, 2 out]
            n144 = property on="On/Off" class="Bool (strict)"("Visible"=w261) -> ()  [unwired: 2 in, 2 out]
            n145 = property on="Test Slider" class="Slide (strict)"("Visible"=w261) -> ()  [unwired: 2 in, 2 out]
          }
          frame "Analog Out", "Motor", "PWM" {
            w267 = FALSE ("Visible")
            n146 = case shown="\"Analog Out\"" w266 {
              tunnel: [1.0 ("Value") -1.0 ("Value") 0.0 ("Value")] -> w265
              tunnel: [255.0 ("Value") 1.0 ("Value") 5.0 ("Value")] -> w264
              tunnel: [128.0 ("Value") 0.0 ("Value") 0.0 ("Value")] -> w263
              tunnel: [64.0 ("Value") 0.5 ("Value") 1.0 ("Value")] -> w262
              frame "PWM" {
              }
              frame "Motor", Default {
              }
              frame "Analog Out" {
              }
            }
            n147 = property on="Motor" class="Clust (strict)"("Visible"=TRUE) -> ()  [unwired: 2 in, 2 out]
            n148 = property on="Value" class="Slide (strict)"("Value"=w263, "Scale.Minimum"=w265, "Scale.Maximum"=w264, "Scale.Increment"=w262) -> ()  [unwired: 2 in, 2 out]
            n149 = property on="On/Off" class="Bool (strict)"("Visible"=w267) -> ()  [unwired: 2 in, 2 out]
            n150 = property on="Test Slider" class="Slide (strict)"("Visible"=w267) -> ()  [unwired: 2 in, 2 out]
            n151 = property on="Test Ring" class="Ring (strict)"("Visible"=w267) -> ()  [unwired: 2 in, 2 out]
            n152 = property on="Rev/Fwd" class="Clust (strict)"("Visible"=w267) -> ()  [unwired: 2 in, 2 out]
          }
          frame "Servo" {
            w283 = FALSE ("Visible")
            n153 = call <vilib>:"NT Read Number.vi"("Name"=w285) -> ("Numeric"=w284:dbl)  [unwired: 9 in, 1 out]
            n154 = property on="Test Slider" class="Slide (strict)"("Visible"=TRUE, "Scale.Maximum"=170.0 ("Scale.Range:Maximum")) -> ()  [unwired: 2 in, 2 out]
            n155 = local write "Test Slider"(w284) -> ()
            n156 = property on="Motor" class="Clust (strict)"("Visible"=w283) -> ()  [unwired: 2 in, 2 out]
            n157 = property on="Rev/Fwd" class="Clust (strict)"("Visible"=w283) -> ()  [unwired: 2 in, 2 out]
            n158 = property on="On/Off" class="Bool (strict)"("Visible"=w283) -> ()  [unwired: 2 in, 2 out]
            n159 = property on="Test Ring" class="Ring (strict)"("Visible"=w283) -> ()  [unwired: 2 in, 2 out]
          }
          frame "Relay", "Solenoid" {
            w286 = FALSE ("Visible")
            n160 = property on="Motor" class="Clust (strict)"("Visible"=w286) -> ()  [unwired: 2 in, 2 out]
            n161 = property on="Test Slider" class="Slide (strict)"("Visible"=w286) -> ()  [unwired: 2 in, 2 out]
            n162 = Search and Replace String(input string=w287, search string="/Value  **", replace string="/Direction") -> (result string=w293:string)  [unwired: 5 in, 3 out]
            n163 = property on="Test Ring" class="Ring (strict)"("Visible"=w286) -> ()  [unwired: 2 in, 2 out]
            n164 = call <vilib>:"NT Read String.vi"("Name"=w293) -> ("String"=w291:string)  [unwired: 9 in, 1 out]
            n165 = Equal?(x="Both directions", y=w291) -> (x = y?=w289:bool)
            n166 = Not(x=w289) -> (.not. x?=w290:bool)
            n167 = property on="Rev/Fwd" class="Clust (strict)"("Visible"=w289) -> ()  [unwired: 2 in, 2 out]
            n168 = property on="On/Off" class="Bool (strict)"("Visible"=w290, "Caption.Text"=w288) -> ()  [unwired: 2 in, 2 out]
          }
          frame "Compressor", "Digital Out" {
            w296 = FALSE ("Visible")
            # "Get direction and finish"
            n169 = property on="Motor" class="Clust (strict)"("Visible"=w296) -> ()  [unwired: 2 in, 2 out]
            n170 = property on="Test Slider" class="Slide (strict)"("Visible"=w296) -> ()  [unwired: 2 in, 2 out]
            n171 = property on="Test Ring" class="Ring (strict)"("Visible"=w296) -> ()  [unwired: 2 in, 2 out]
            n172 = property on="On/Off" class="Bool (strict)"("Visible"=TRUE, "Caption.Text"=w297) -> ()  [unwired: 2 in, 2 out]
            n173 = property on="Rev/Fwd" class="Clust (strict)"("Visible"=FALSE) -> ()  [unwired: 2 in, 2 out]
          }
          frame "Camera" {
            n174 = call <vilib>:"Get Last Path Segment.vi"("String in"=w304) -> ("String out"=w305:string)  [unwired: 10 in]
            n175 = property on="On/Off" class="Bool (strict)"("Visible"=FALSE) -> ()  [unwired: 2 in, 2 out]
            n176 = property on="Motor" class="Clust (strict)"("Visible"=FALSE) -> ()  [unwired: 2 in, 2 out]
            n177 = property on="Rev/Fwd" class="Clust (strict)"("Visible"=FALSE) -> ()  [unwired: 2 in, 2 out]
            n178 = case shown="\"White Balance  **\"" w305 {
              tunnel: w304 -> [w311 w320 w329 w338 w347 _ w353]
              tunnel: w303 -> [w309 w317 w326 w335 w344 _ _]
              frame "Size  **" {
                n179 = Index Array(array=w309) -> (element=w308:cluster{string[]})  [unwired: 1 in]
                n180 = call <vilib>:"NT Read String.vi"("Name"=w311) -> ("String"=w310:string)  [unwired: 9 in, 1 out]
                n181 = Unbundle(w308) -> (w306:string[])
                n182 = Match First String(2:w306, 3:w310) -> (0:w307:i32)  [unwired: 1 out]
                n183 = property on="Test Ring" class="Ring (strict)"("Value"=w307, "Strings []"=w306) -> ()  [unwired: 2 in, 2 out]
                n184 = property on="Test Ring" class="Ring (strict)"("Visible"=TRUE) -> ()  [unwired: 2 in, 2 out]
                n185 = property on="Test Slider" class="Slide (strict)"("Visible"=FALSE) -> ()  [unwired: 2 in, 2 out]
              }
              frame "White Balance  **" {
                n186 = Index Array(array=w317, index=1) -> (element=w318:cluster{string[]})
                n187 = call <vilib>:"NT Read String.vi"("Name"=w320) -> ("String"=w319:string)  [unwired: 9 in, 1 out]
                n188 = Unbundle(w318) -> (w315:string[])
                n189 = Match First String(2:w315, 3:w319) -> (0:w314:i32)  [unwired: 1 out]
                n190 = property on="Test Ring" class="Ring (strict)"("Value"=w314, "Strings []"=w315) -> ()  [unwired: 2 in, 2 out]
                n191 = property on="Test Ring" class="Ring (strict)"("Visible"=TRUE) -> ()  [unwired: 2 in, 2 out]
                n192 = property on="Test Slider" class="Slide (strict)"("Visible"=FALSE) -> ()  [unwired: 2 in, 2 out]
              }
              frame "Exposure  **" {
                n193 = Index Array(array=w326, index=2) -> (element=w327:cluster{string[]})
                n194 = call <vilib>:"NT Read String.vi"("Name"=w329) -> ("String"=w328:string)  [unwired: 9 in, 1 out]
                n195 = Unbundle(w327) -> (w323:string[])
                n196 = Match First String(2:w323, 3:w328) -> (0:w324:i32)  [unwired: 1 out]
                n197 = property on="Test Ring" class="Ring (strict)"("Value"=w324, "Strings []"=w323) -> ()  [unwired: 2 in, 2 out]
                n198 = property on="Test Ring" class="Ring (strict)"("Visible"=TRUE) -> ()  [unwired: 2 in, 2 out]
                n199 = property on="Test Slider" class="Slide (strict)"("Visible"=FALSE) -> ()  [unwired: 2 in, 2 out]
              }
              frame "Exposure Priority  **" {
                n200 = Index Array(array=w335, index=3) -> (element=w336:cluster{string[]})
                n201 = call <vilib>:"NT Read String.vi"("Name"=w338) -> ("String"=w337:string)  [unwired: 9 in, 1 out]
                n202 = Unbundle(w336) -> (w332:string[])
                n203 = Match First String(2:w332, 3:w337) -> (0:w333:i32)  [unwired: 1 out]
                n204 = property on="Test Ring" class="Ring (strict)"("Value"=w333, "Strings []"=w332) -> ()  [unwired: 2 in, 2 out]
                n205 = property on="Test Ring" class="Ring (strict)"("Visible"=TRUE) -> ()  [unwired: 2 in, 2 out]
                n206 = property on="Test Slider" class="Slide (strict)"("Visible"=FALSE) -> ()  [unwired: 2 in, 2 out]
              }
              frame "Color Enable  **" {
                n207 = Index Array(array=w344, index=4) -> (element=w345:cluster{string[]})
                n208 = call <vilib>:"NT Read String.vi"("Name"=w347) -> ("String"=w346:string)  [unwired: 9 in, 1 out]
                n209 = Unbundle(w345) -> (w341:string[])
                n210 = Match First String(2:w341, 3:w346) -> (0:w342:i32)  [unwired: 1 out]
                n211 = property on="Test Ring" class="Ring (strict)"("Value"=w342, "Strings []"=w341) -> ()  [unwired: 2 in, 2 out]
                n212 = property on="Test Ring" class="Ring (strict)"("Visible"=TRUE) -> ()  [unwired: 2 in, 2 out]
                n213 = property on="Test Slider" class="Slide (strict)"("Visible"=FALSE) -> ()  [unwired: 2 in, 2 out]
              }
              frame Default {
                n214 = property on="Test Ring" class="Ring (strict)"("Visible"=FALSE) -> ()  [unwired: 2 in, 2 out]
                n215 = property on="Test Slider" class="Slide (strict)"("Visible"=FALSE) -> ()  [unwired: 2 in, 2 out]
              }
              frame "Brightness  **", "Color Level  **", "Compression  **", "FPS  **", "Sharpness  **" {
                n216 = call <vilib>:"NT Read Number.vi"("Name"=w353) -> ("Numeric"=w352:dbl)  [unwired: 9 in, 1 out]
                n217 = local write "Test Slider"(w352) -> ()
                n218 = property on="Test Slider" class="Slide (strict)"("Visible"=TRUE, "Scale.Maximum"=100.0 ("Scale.Range:Maximum")) -> ()  [unwired: 2 in, 2 out]
                n219 = property on="Test Ring" class="Ring (strict)"("Visible"=FALSE) -> ()  [unwired: 2 in, 2 out]
              }
            }
          }
        }
      }
      event "Test Name": Mouse Enter {
        # "Populate the ring with the list of tests"
        n220 = event-data() -> ()  [unwired: 1 in, 1 out]
        n221 = call <vilib>:"NT Read String Array.vi"("Name"="TestMode/TestList") -> ("String Array"=w361:string[])  [unwired: 9 in, 1 out]
        n222 = Build Array (concatenate)("Select the test to run...", w361) -> (w360:string[])
        n223 = property on="Test Name" class="Ring (strict)"("Strings []"=w360) -> ()  [unwired: 2 in, 2 out]
      }
      event "Test Name": Value Change {
        w363 = FALSE ("Visible")
        # "Tell the robot the test name to run"
        n224 = event-data() -> ("NewVal"=w367:u16)  [unwired: 1 in]
        n225 = property on="Test Name" class="Ring (strict)"() -> ("Strings []"=w368:string[])  [unwired: 2 in, 2 out]
        n226 = local write "Progress"(T6 {"Test Progress"=0, "Test Progress Text"=""} ("Progress")) -> ()
        n227 = Index Array(array=w368, index=w367) -> (element=w366:string)
        n228 = call <vilib>:"NT Write String.vi"("String"=w366, "Name"="TestMode/TestName") -> ()  [unwired: 9 in, 1 out]
        n229 = property on="Progress" class="Clust (strict)"("Visible"=TRUE) -> ()  [unwired: 2 in, 2 out]
        n230 = property on="Motor" class="Clust (strict)"("Visible"=w363) -> ()  [unwired: 2 in, 2 out]
        n231 = property on="Test Slider" class="Slide (strict)"("Visible"=w363) -> ()  [unwired: 2 in, 2 out]
        n232 = property on="On/Off" class="Bool (strict)"("Visible"=w363) -> ()  [unwired: 2 in, 2 out]
        n233 = property on="Rev/Fwd" class="Clust (strict)"("Visible"=w363) -> ()  [unwired: 2 in, 2 out]
        n234 = property on="Test Ring" class="Ring (strict)"("Visible"=w363) -> ()  [unwired: 2 in, 2 out]
      }
      event "Select Auto": Mouse Enter {
        # "Populate the combo box with the list of autonomous options"
        n235 = event-data() -> ()  [unwired: 1 in, 1 out]
        n236 = call <vilib>:"NT Read String Array.vi"("Name"="Auto List") -> ("String Array"=w370:string[])  [unwired: 9 in, 1 out]
        n237 = property on="Select Auto" class="CmbBox"("Strings[]"=w370) -> ()  [unwired: 2 in, 2 out]
      }
      event "Select Auto": Value Change {
        # "User modified the Auto Selection. Write to NT variable so robot knows."
        n238 = event-data() -> ("NewVal"=w373:string)  [unwired: 1 in]
        n239 = call <vilib>:"NT Write String.vi"("String"=w373, "Name"="Auto Selector") -> ()  [unwired: 9 in, 1 out]
      }
      event "Command Selection": Value Change {
        # "Get the params and show in table"
        n240 = event-data() -> ("NewVal"=w379:i32)  [unwired: 1 in]
        n241 = property on="Command Selection" class="MCListbox (strict)"() -> ("ItemNames"=w377:string[][])  [unwired: 2 in, 2 out]
        n242 = call <vilib>:"WPI_DashboardUpdate Command Params.vi"("NewVal"=w379, "Commands"=w377, "Param Tbl"=w378) -> ()  [unwired: 8 in, 1 out]
      }
      event "Execute Command": Value Change {
        # "Started one, Unique ID holds\nresponse"
        n243 = event-data() -> ()  [unwired: 1 in, 1 out]
        n244 = property on="Command Selection" class="MCListbox (strict)"() -> ("ItemNames"=w390:string[][])  [unwired: 2 in, 2 out]
        n245 = Index Array(array=w390, index (row)="Command Selection", index (col)=0) -> (element=w388:string)
        n246 = call <vilib>:"Invoke Commands.vi"("Command Params"="Command Params", "Function Name"=w388) -> ("Params"=w384:u8, "Started"=w383:bool)  [unwired: 7 in, 1 out]
        n247 = Array Subset(array="Command Params", length (row)=w384) -> (w385:string[][])  [unwired: 3 in]
        n248 = Select(t="Executing" ("Cmd Status"), s=w383, f="" ("Cmd Status")) -> (s? t:f=→"Cmd Status":string)
      }
      event "Command Selection": Double Click {
        n249 = event-data() -> ("Row"=w398:i32)  [unwired: 1 in]
        n250 = property on="Command Selection" class="MCListbox (strict)"() -> ("ItemNames"=w401:string[][])  [unwired: 2 in, 2 out]
        n251 = local read "Command Params"() -> (w397:string[][])
        n252 = Index Array(array=w401, index (row)=w398, index (col)=0) -> (element=w399:string)
        n253 = call <vilib>:"Invoke Commands.vi"("Command Params"=w397, "Function Name"=w399) -> ("Params"=w396:u8, "Started"=w391:bool)  [unwired: 7 in, 1 out]
        n254 = Array Subset(array=w397, length (row)=w396) -> (w395:string[][])  [unwired: 3 in]
        n255 = Select(t="Executing" ("Cmd Status"), s=w391, f="" ("Cmd Status")) -> (s? t:f=w392:string)
        n256 = local write "Cmd Status"(w392) -> ()
      }
      event "CheckList": Double Click {
        # "Shift clears all"
        # "Update symbols on the listbox"
        n257 = event-data() -> ("PlatMods.Shift"=w403:bool, "Row"=w405:i32)  [unwired: 1 in]
        n258 = case shown="True" w403 {
          tunnel: w405 -> [w409 _]
          tunnel: 1 -> [w408 _]
          frame False {
            n259 = property on="CheckList" class="LstBox (strict)"() -> ("Item Symbols"=w407:i32[])  [unwired: 2 in, 2 out]
            n260 = Replace Array Subset(array=w407, new element=w408, index=w409) -> (w406:i32[])
            n261 = property on="CheckList" class="LstBox (strict)"("Item Symbols"=w406) -> ()  [unwired: 2 in, 2 out]
          }
          frame True {
            w410 = 0 ("Top Row")
            n262 = property on="CheckList" class="LstBox (strict)"() -> ("Number of Rows"=w412:u32)  [unwired: 2 in, 2 out]
            n263 = Initialize Array(0, w412) -> (w411:i32[])
            n264 = property on="CheckList" class="LstBox (strict)"("Top Row"=w410, "Value"=w410, "Item Symbols"=w411) -> ()  [unwired: 2 in, 2 out]
          }
        }
      }
      event "CheckList": Key Down {
        # "Update symbols on the listbox\nLeft and right keys check and uncheck"
        n265 = event-data() -> ("VKey"=w416:T23)  [unwired: 1 in]
        n266 = case shown="\"Left\", \"Right\"" w416 {
          selector: w416 -> [w421 _]
          tunnel: eventvkey."Left" ("VKey") -> [w419 _]
          frame "Left", "Right" {
            n267 = Equal?(x=w419, y=w421) -> (x = y?=w420:bool)
            n268 = Select(t=0, s=w420, f=1) -> (s? t:f=w422:i32)
            n269 = property on="CheckList" class="LstBox (strict)"() -> ("Item Symbols"=w425:i32[])  [unwired: 2 in, 2 out]
            n270 = Replace Array Subset(array=w425, new element=w422, index="CheckList") -> (w424:i32[])
            n271 = property on="CheckList" class="LstBox (strict)"("Item Symbols"=w424) -> ()  [unwired: 2 in, 2 out]
          }
          frame Default {
          }
        }
      }
      event "Motor.Enable": Value Change {
        # "When the test mode otor enable helper is set, update that\ntree row item's value"
        n272 = event-data() -> ("NewVal"=w431:bool)  [unwired: 1 in]
        n273 = Unbundle("Motor") -> ("Value"=w430:dbl)  [unwired: 1 out]
        n274 = Select(t=w430, s=w431, f=0.0) -> (s? t:f=w428:dbl)
        n275 = call <vilib>:"NT Write Number.vi"("Numeric"=w428, "Name"=w427) -> ()  [unwired: 9 in, 1 out]
      }
      event "Test Slider": Value Change {
        # "When the test mode slider helper is set, update that\ntree row item's value"
        n276 = event-data() -> ("NewVal"=w434:dbl)  [unwired: 1 in]
        n277 = call <vilib>:"NT Write Number.vi"("Numeric"=w434, "Name"=w435) -> ()  [unwired: 9 in, 1 out]
      }
      event "On/Off": Value Change {
        # "When the test mode on/off helper value is set, update that\ntree row item's value"
        n278 = event-data() -> ("NewVal"=w439:bool)  [unwired: 1 in]
        n279 = Boolean To (0,1)(Boolean=w439) -> (0, 1=w438:i16)
        n280 = call <vilib>:"NT Write Number.vi"("Numeric"=w438, "Name"=w437) -> ()  [unwired: 9 in, 1 out]
      }
      event "Rev/Fwd": Value Change {
        # "When the test mode helper value for relays is set, update that\ntree row item's value"
        n281 = event-data() -> ("NewVal.Forward"=w447:bool, "NewVal.Reverse"=w446:bool)  [unwired: 1 in]
        n282 = Boolean To (0,1)(Boolean=w447) -> (0, 1=w443:i16)
        n283 = Boolean To (0,1)(Boolean=w446) -> (0, 1=w445:i16)
        n284 = Negate(x=w445) -> (-x=w444:i16)
        n285 = Add(x=w443, y=w444) -> (x+y=w442:i16)
        n286 = call <vilib>:"NT Write Number.vi"("Numeric"=w442, "Name"=w441) -> ()  [unwired: 9 in, 1 out]
      }
      event "Test Ring": Value Change {
        # "When a test mode helper value is selected from the ring,\nset the tree item's variable to the string value"
        n287 = event-data() -> ("NewVal"=w451:u16)  [unwired: 1 in]
        n288 = property on="Test Ring" class="Ring (strict)"() -> ("Strings []"=w452:string[])  [unwired: 2 in, 2 out]
        n289 = Index Array(array=w452, index=w451) -> (element=w450:string)
        n290 = call <vilib>:"NT Write String.vi"("String"=w450, "Name"=w449) -> ()  [unwired: 9 in, 1 out]
      }
      event "Rec Mode": Value Change {
        # "Update globals for recording mode and path to read log from.\nClear when logging and let NetworkTables set path for vision to\nuse."
        n291 = event-data() -> ("NewVal"=w463:enum32{"Stop", "Record", "Playback"})  [unwired: 1 in]
        n292 = global write "WPI_DashboardLogging Global.vi" "Logging Filename"(path "") -> ()
        n293 = global write "WPI_DashboardLogging Global.vi" "Recording"(w463) -> ()
        n294 = case shown="\"Playback\"" w463 {
          tunnel: w462 -> [_ w465 w474]
          tunnel: [_ _ w473] -> w460
          tunnel: [_ _ w472] -> _
          tunnel: w458 -> [_ _ w470]
          tunnel: cluster{i32, i32} {-250, 170} -> [_ _ w469]
          tunnel: [_ _ T24 {"Image Size"=TRUE, "Image Type"=TRUE, "Pixel Value"=TRUE, "ROI Information"=TRUE, "Zoom Factor"=FALSE} ("Image Information Shown:All Elements")] -> w453
          tunnel: [_ _ TRUE ("Zoom Factor")] -> w454
          tunnel: w456 -> [_ _ w466]
          frame Default {
          }
          frame "Stop", "Record" {
            # "Place Window too"
            n295 = invoke class="VI" method="FP.Close"(reference=w465) -> (reference out=w464:refnum<vi>)  [unwired: 2 in, 2 out]
            n296 = invoke class="VI" method="Abort VI"(reference=w464) -> ()  [unwired: 2 in, 3 out]
          }
          frame "Playback" {
            n297 = call "Open Playback Panel.vi"("Offset"=w469, "DB VI Ref"=w470, "Playback in"=w474) -> ("Playback out"=w471:refnum<vi>)  [unwired: 8 in]
            n298 = register-events(w471, w466) -> (reference out=w473:refnum<event-registration>, error out=w472:errorcluster)  [unwired: 2 in]
          }
        }
        n299 = property on="Camera Image Right" class="ImageControl"("Image Information Shown"=w453, "Image Information Visible"=w454) -> ()  [unwired: 2 in, 2 out]
        n300 = property on="Camera Image" class="ImageControl"("Image Information Shown"=w453, "Image Information Visible"=w454) -> ()  [unwired: 2 in, 2 out]
        n301 = call <vilib>:"WPI_DashboardNT Log FieldName Cache.vi"("Operation"=enum16{"Lookup/Add", "Index", "Clear"}."Clear") -> ()  [unwired: 8 in, 3 out]
      }
      event Panel Close {
        w476 = enum32{"Stop", "Record", "Playback"}."Stop" ("Rec Mode")
        # "Playback window has been closed, abort"
        n302 = event-data() -> ()  [unwired: 1 in, 4 out]
        n303 = local write "Rec Mode"(w476) -> ()
        n304 = global write "WPI_DashboardLogging Global.vi" "Recording"(w476) -> ()
      }
      event Panel Close {
        # "Abort playback window and ourself"
        n305 = event-data() -> ()  [unwired: 1 in, 4 out]
        n306 = invoke class="VI" method="FP.Close"(reference=w480) -> (reference out=w479:refnum<vi>)  [unwired: 2 in, 2 out]
        n307 = invoke class="VI" method="Abort VI"(reference=w479) -> (error out=w478:errorcluster)  [unwired: 2 in, 2 out]
        n308 = invoke class="VI" method="Abort VI"(error in=w478) -> ()  [unwired: 2 in, 3 out]
      }
      event User Event {
        n309 = event-data() -> ("IDs"=w487:cluster{"RPC field ID":u16, "Unique ID":u16}, "String"=w486:string)  [unwired: 1 in]
        n310 = Bundle("IDs"=w487, "String"=w486) -> (w485:T10)  [unwired: 1 in]
        n311 = call <vilib>:"Retrieve RPC Response.vi"("RPC Response"=w485) -> ("Output"=w483:string[][])  [unwired: 10 in]
        n312 = Build Array (concatenate)(w481, w483) -> (w482:string[][])
        n313 = local write "Command Params"(w482) -> ()
        n314 = local write "Cmd Status"("" ("Cmd Status")) -> ()
      }
      event "Tree": Double Click {
        n315 = event-data() -> ("PlatMods"=w493:T27, "Tag"=w490:string)  [unwired: 1 in]
        n316 = Unbundle(w493) -> ("Shift"=w492:bool)  [unwired: 4 out]
        n317 = String Subset(string=w490, length (rest)=1 ("length (rest)")) -> (substring=w489:string)  [unwired: 1 in]
        n318 = Not(x=w492) -> (.not. x?=w491:bool)
        n319 = case shown="\"/\"" w489 {
          tunnel: w490 -> [_ w496]
          tunnel: w491 -> [_ w495]
          frame Default {
          }
          frame "/" {
            n320 = call <vilib>:"NT Update Persistence.vi"("Persistence"=w495, "Name"=w496) -> ()  [unwired: 9 in, 1 out]
          }
        }
      }
    }
  }
  n321 = while {
    tunnel: w65 -> [w498]
    i -> [w501]
    stop <- FALSE stop-if-true
    n322 = Wait (ms)(milliseconds to wait=u32 100) -> ()  [unwired: 1 out]
    n323 = case shown="\"Playback\"" "Rec Mode" {
      tunnel: w501 -> [_ _ w516]
      tunnel: [u32 2829099 ("Base Color") u32 11141120 ("Target Color") w505] -> w497
      frame "Stop", Default {
        # "Reset the color, extra updates don't cost much"
      }
      frame "Record" {
      }
      frame "Playback" {
        # "Playback"
        n324 = Quotient & Remainder(x=w516, y=u32 50 ("milliseconds to wait")) -> (x-y*floor(x/y)=w512:u32)  [unwired: 1 out]
        n325 = Divide(x=w512, y=u32 50 ("milliseconds to wait")) -> (x/y=w509:dbl)
        n326 = Multiply(x=6.283185307179586, y=w509) -> (x*y=w514:dbl)
        n327 = Sine(x=w514) -> (sin(x)=w513:dbl)
        n328 = Absolute Value(x=w513) -> (abs(x)=w506:dbl)
        n329 = call "Interpolate RGB Color.vi"("Proportion"=w506, "Target Color"=u32 30976, "Base Color"=u32 2829099) -> ("Result Color"=w505:u32)  [unwired: 8 in]
      }
    }
    n330 = property class="Pane"(reference=w498, "PaneColor"=w497) -> ()  [unwired: 1 in, 2 out]
  }
  n331 = local write "Dashboard Tab"(T2."Drive" ("Dashboard Tab")) -> ()
  n332 = property on="On/Off" class="Bool (strict)"("Visible"=w36) -> ()  [unwired: 2 in, 2 out]
  n333 = property on="Motor" class="Clust (strict)"("Visible"=w36) -> ()  [unwired: 2 in, 2 out]
  n334 = property on="Progress" class="Clust (strict)"("Visible"=w36) -> ()  [unwired: 2 in, 2 out]
  n335 = property on="Test Ring" class="Ring (strict)"("Visible"=w36) -> ()  [unwired: 2 in, 2 out]
  n336 = property on="Rev/Fwd" class="Clust (strict)"("Visible"=w36) -> ()  [unwired: 2 in, 2 out]
  n337 = while {
    tunnel: u16 1741 ("timeout ms (25000)") -> [w518]
    stop <- FALSE stop-if-true
    n338 = TCP Create Listener(10:w518) -> (0:w517:errorcluster, 3:w519:refnum<k5>)  [unwired: 4 in, 1 out]
    n339 = case shown="No Error" w517 {
      selector: w517 -> [w521 _]
      tunnel: w519 -> [w522 _]
      frame No Error {
        n340 = while {
          tunnel: w522 -> [w525]
          tunnel: w521 -> [w524]
          stop <- FALSE stop-if-true
          n341 = TCP Wait On Listener(8:w524, 11:w525) -> (0:w526:errorcluster, 4:w527:refnum<k5>)  [unwired: 2 in, 3 out]
          n342 = local write "TCP"(w527) -> ()
          n343 = case shown="No Error" w526 {
            frame No Error {
            }
            frame Error {
              n344 = Wait (ms)(milliseconds to wait=u32 1000) -> ()  [unwired: 1 out]
            }
          }
        }
      }
      frame Error {
        n345 = Wait (ms)(milliseconds to wait=u32 1000) -> ()  [unwired: 1 out]
      }
    }
  }
  n346 = local write "Command Selection"(u16 0 ("milliseconds to wait")) -> ()
  n347 = local write "Command Params"(string[][] [] ("Command Params")) -> ()
  n348 = global write "WPI_DashboardLogging Global.vi" "Recording"(w59) -> ()
  n349 = local write "Rec Mode"(w59) -> ()
  n350 = call <vilib>:"NT Write String.vi"("String"="Select Auto", "Name"="Auto Selector") -> ()  [unwired: 9 in, 1 out]
